vi "Drivetrain Loop.vi"() -> ()   [LabVIEW 2013]
uses:
  DT Mode.ctl
  Drivetrain Status.ctl
  Common Code/Change Detect Int.vi
  Robot Global Data.vi
  <vilib>/Rock Robotics/WPI/Solenoid/Deprecated/WPI_SolenoidSetBool.vi
  <vilib>/Rock Robotics/WPI/AnalogModule/WPI_AnalogModuleGetAverageVoltage.vi
  <vilib>/Utility/error.llb/Clear Errors.vi
panel:
  out "Mode":T1
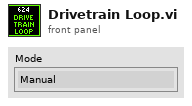
[diagram p1: front panel]
types:
  T1 = typedef "DT Mode.ctl" = enum16{"Manual", "Gyro Steer", "Distance Drive", "Fieldcentric", "Roll Maneuver", "Alt Roll Maneuver"}
  T2 = typedef "Drivetrain Status.ctl" = cluster{"Mode":T1, "X":dbl, "Y":dbl, "Steer":dbl, "Low Gear":bool, "Omni":bool}
  T3 = typedef "Drivetrain Control.ctl" = cluster{"axis 1 (x)":dbl, "axis 2 (y)":dbl, "Mode":T1, "heading target":dbl, "steer axis":dbl, "omni?":bool, "Low Gear?":bool, "distance target":cluster{"x":dbl, "y":dbl}, "PID Params":cluster{"X Dist":cluster{"PID gains":cluster{"proportional gain (Kc)":dbl, "integral time (Ti, min)":dbl, "derivative time (Td, min)":dbl}, "output range":cluster{"output high":dbl, "output low":dbl}}, "Y Dist":cluster{"PID gains":cluster{"proportional gain (Kc)":dbl, "integral time (Ti, min)":dbl, "derivative time (Td, min)":dbl}, "output range":cluster{"output high":dbl, "output low":dbl}}}, "Coast":bool}
  T4 = typedef "WPI_DriverStationRobotMode2.ctl" = enum16{"Autonomous Disabled", "Autonomous Enabled", "Teleop Disabled", "Teleop Enabled", "Timeout", "Finish", "Test Disabled", "Test Enabled"}
  T5 = typedef "Dashboard UDP Packet.ctl" = cluster{"Camera":T6, "Gyro":T7, "Encoder":T9, "Auto Shift":T10, "Auton":T11, "Drive/Ramp X":dbl, "Drive/Ramp Y":dbl, "Drive/Battery Cutoff":dbl, "Pressure/Compressor Min Voltage":dbl, "Pressure/Compressor Delay":dbl, "Controller/Strafe Correction":bool, "Shooter":T12, "Rollers":T13, "Abort":bool, "Finish":bool, "IR Halo Sustain Time":dbl, "Disable Compressor":bool, "Center Omni Drive Delay":i32, "Vision Mode":T14, "Radius Throttle":bool, "Fieldcentric":T15, "Roll":T16, "Stick Deadband":dbl}
  T6 = typedef "Camera Controls.ctl" = cluster{"Camera/View Angle X":dbl, "Camera/Goal Track Timeout":dbl, "Camera/View Angle Y":dbl, "Camera/Goal Exposure":dbl, "Camera/Vision Receive Timeout":dbl, "Camera/Offset 1":dbl, "Camera/Offset 2":dbl}
  T7 = typedef "Gyro Controls.ctl" = cluster{"Gyro/Angle Tolerance":dbl, "Gyro/Steer Closeness Threshold":dbl, "Steer PID":T8, "Steer Close PID":T8}
  T8 = typedef "PID Params.ctl" = cluster{"max":dbl, "min":dbl, "P":dbl, "I":dbl, "D":dbl}
  T9 = typedef "Encoder Controls.ctl" = cluster{"Encoders/Reset":bool, "Encoders/Omni Constant":dbl, "Encoders/Omni Tick Constant":dbl, "Encoders/Left Constant":dbl, "Encoders/Right Constant":dbl, "Encoders/Right Tick Constant":dbl}
  T10 = typedef "Auto Shift Controls.ctl" = cluster{"AutoShift/Upshift Throttle Accel":dbl, "AutoShift/Speed Threshold":dbl, "AutoShift/Upshift Throttle":dbl, "AutoShift/Upshift Accel":dbl, "AutoShift/Downshift Accel":dbl, "AutoShift/Downshift Throttle":dbl, "AutoShift/Delay":dbl, "AutoShift/Enabled":bool}
  T11 = typedef "Auton Controls.ctl" = cluster{"Auton/Left Shoot X-Coord":dbl, "Auton/Right Shoot X-Coord":dbl, "DistDrive/Distance Stop Threshold":dbl, "DistDrive/Max Stop Speed":dbl, "Auton/Back Piston Time":dbl, "Auton/Manual Hot":bool, "Auton/Manual Hot Right":bool, "Default X PID":T8, "Default Y PID":T8}
  T12 = typedef "Shooter Controls.ctl" = cluster{"Shooter/Reset Time":dbl, "Shooter/Release Delay":dbl, "Shooter/Pressure Steady Time":dbl, "Shooter/Misfire Delay":dbl, "Shooter/Ball Settle Time":dbl, "Shooter/Line IR Delay":dbl, "Pressure/Upper PSI Time":dbl, "Pressure/Lower PSI Time":dbl, "Shooter/Punch Delay":dbl, "Shooter/Target Pressure":dbl, "Pressure/Line B":dbl, "Pressure/Line M":dbl, "Pressure/Shooter M":dbl, "Pressure/Shooter B":dbl, "Halo Time":dbl, "Soft Release Delay":dbl, "Soft Unpin Delay":dbl, "Soft Shoot Delay":dbl}
  T13 = typedef "Roller Controls.ctl" = cluster{"Roller/Load IRs Verify Time":dbl, "Roller/Center IR Latch Time":dbl, "Roller/Speed Front":dbl, "Roller/Speed Back":dbl, "Roller/Entry Timeout":dbl, "Roller/To Center Timeout":dbl, "Roller/Sustain Time":dbl, "Roller/Verify Center Time":dbl}
  T14 = typedef "Vision Mode.ctl" = enum16{"Normal", "Extreme Left", "Extreme Right"}
  T15 = typedef "Fieldcentric Controls.ctl" = cluster{"Relative Angle":bool, "Point Robot":bool, "X/Y ratio low":dbl, "Steering Gain":dbl, "Force Omni Down":bool, "Enable":bool, "X/Y ratio high":dbl}
  T16 = typedef "Roll Maneuver.ctl" = cluster{"X 1":dbl, "Y 1":dbl, "Y 2":dbl, "X 2":dbl, "Y 3":dbl, "X 3":dbl, "Time 1":i32, "Time 2":i32, "Time 3":i32, "Angle Start":dbl, "Angle End":dbl, "Angle Linearity":dbl}
  T17 = cluster{"X Dist":cluster{"PID gains":cluster{"proportional gain (Kc)":dbl, "integral time (Ti, min)":dbl, "derivative time (Td, min)":dbl}, "output range":cluster{"output high":dbl, "output low":dbl}}, "Y Dist":cluster{"PID gains":cluster{"proportional gain (Kc)":dbl, "integral time (Ti, min)":dbl, "derivative time (Td, min)":dbl}, "output range":cluster{"output high":dbl, "output low":dbl}}}
  T18 = typedef "WPI_SolenoidDevRef.ctl" = cluster{"DevStatus":errorcluster, "Solenoid Module":T19, "Forward Solenoid Channel":T20, "Reverse Solenoid Channel":T20}
  T19 = typedef "FPGA_TypedefSolenoidModule.ctl" = enum16{"Solenoid Module 1", "Solenoid Module 2"}
  T20 = typedef "WPI_SolenoidChannel.ctl" = enum8{"Solenoid 1", "Solenoid 2", "Solenoid 3", "Solenoid 4", "Solenoid 5", "Solenoid 6", "Solenoid 7", "Solenoid 8", "Invalid"}
  T21 = typedef "WPI_MotorControlDeviceRef.ctl" = cluster{"DeviceStatus":errorcluster, "Type":enum16{"PWM", "CAN"}, "PWM":cluster{"Digital Module":T22, "PWM Channel":T23, "DeadBand":T24}, "CAN":cluster{"Device Number":u8, "Control Mode":T25, "Semaphore":T26, "Max Vout":dbl}, "Invert":bool, "TransformRef":T27, "InvTransformRef":T27}
  T22 = typedef "FPGA_TypedefDigitalModule.ctl" = enum16{"Digital Module 1", "Digital Module 2"}
  T23 = typedef "FPGA_DIOPWMChannel.ctl" = enum8{"PWM 1", "PWM 2", "PWM 3", "PWM 4", "PWM 5", "PWM 6", "PWM 7", "PWM 8", "PWM 9", "PWM 10", "Invalid"}
  T24 = typedef "WPI_PWMDeadband.ctl" = cluster{"Name":string, "maxPositivePwm":i32, "minPositivePwm":i32, "centerPwm":i32, "maxNegativePwm":i32, "minNegativePwm":i32, "angularRange":u16}
  T25 = typedef "WPI_CANJaguar_ControlMode.ctl" = enum8{"Percent VBus", "Current", "Speed", "Position", "Voltage"}
  T26 = typedef "Semaphore RefNum" = refnum<k1>
  T27 = typedef "WPI_PWMTransform_ConPane.ctl" = refnum<vi>
  T28 = typedef "Arcade Drive Ref.ctl" = cluster{"L1":T21, "L2":T21, "R1":T21, "R2":T21, "Motor Count":enum16{"2 Motor", "4 Motor"}, "L Reversed?":bool, "R Reversed?":bool}
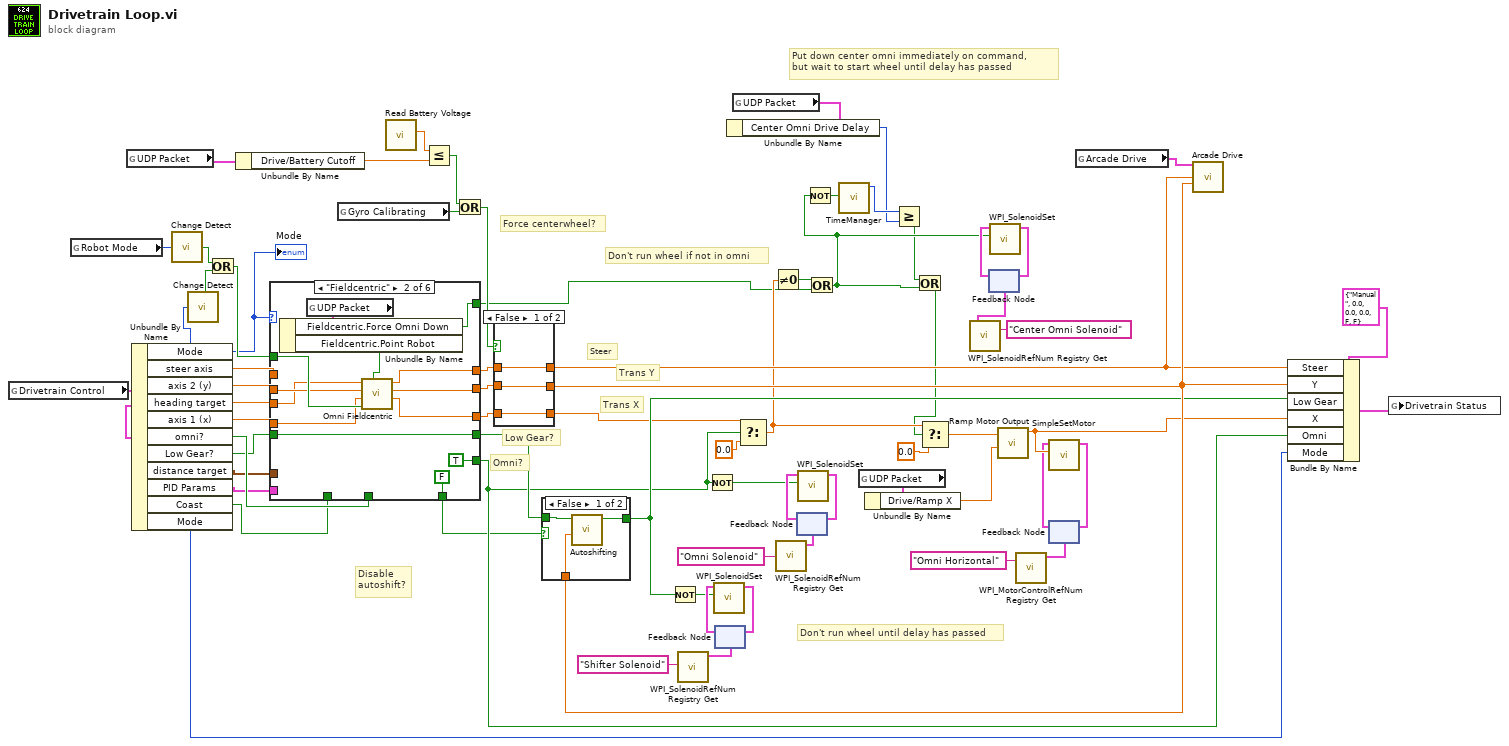
[diagram p0: block diagram]
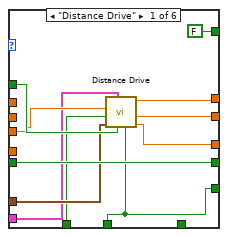
[diagram p3: hidden frame]
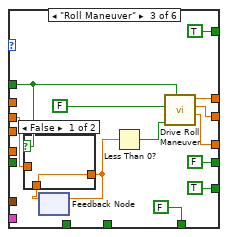
[diagram p4: hidden frame]
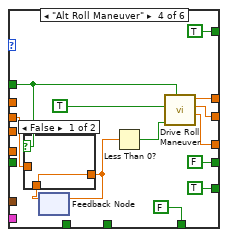
[diagram p6: hidden frame]
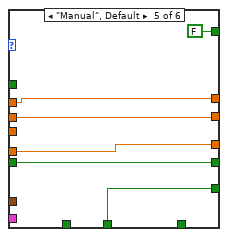
[diagram p8: hidden frame]
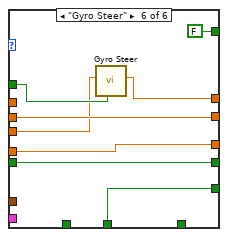
[diagram p9: hidden frame]
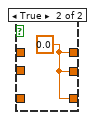
[diagram p10: hidden frame]
diagram:
  # "Disable \nautoshift?"
  # "Force centerwheel?"
  # "Don't run wheel until delay has passed"
  # "Don't run wheel if not in omni"
  # "Put down center omni immediately on command,\nbut wait to start wheel until delay has passed"
  # "Low Gear?"
  # "Omni?"
  # "Trans X"
  # "Steer"
  # "Trans Y"
  n1 = global read "Robot Global Data.vi" "Drivetrain Control"() -> (w51:T3)
  n2 = global read "Robot Global Data.vi" "Robot Mode"() -> (w67:T4)
  n3 = global read "Robot Global Data.vi" "UDP Packet"() -> (w45:T5)
  n4 = Unbundle By Name(w51) -> ("Mode"=w60:T1, "steer axis"=w59:dbl, "axis 2 (y)"=w58:dbl, "heading target"=w57:dbl, "axis 1 (x)"=w56:dbl, "omni?"=w55:bool, "Low Gear?"=w54:bool, "distance target"=w53:cluster{"x":dbl, "y":dbl}, "PID Params"=w52:T17, "Coast"=w46:bool, "Mode"=w1:T1)
  "Mode" <- w60
  n5 = call-poly "Change Detect.vi"("In"=w67) -> ("Changed?"=w68:bool)
  n6 = call-poly "Change Detect.vi"("In"=w60) -> ("Changed?"=w69:bool)
  n7 = Or(x=w68, y=w69) -> (x .or. y?=w63:bool)
  n8 = Unbundle By Name(w45) -> ("Drive/Battery Cutoff"=w44:dbl)
  n9 = case shown="\"Fieldcentric\"" w60 {
    tunnel: w59 -> [_ _ _ _ w129 _]
    tunnel: [w76 w87 w106 w121 w129 w133] -> w66
    tunnel: w58 -> [_ w91 w97 w112 w128 w137]
    tunnel: [w77 w88 w105 w120 w128 w137] -> w65
    tunnel: w63 -> [w75 w93 w98 w113 _ w132]
    tunnel: w57 -> [w74 w90 _ _ _ w131]
    tunnel: [w78 w89 w104 w119 w127 w136] -> w64
    tunnel: w56 -> [_ w92 _ _ w127 w136]
    tunnel: w55 -> [w79 _ _ _ w125 w134]
    tunnel: w54 -> [w80 w81 _ _ w126 w135]
    tunnel: w52 -> [w72 _ _ _ _ _]
    tunnel: w53 -> [w73 _ _ _ _ _]
    tunnel: [w80 w81 FALSE ("Low Gear?") FALSE ("Low Gear?") w126 w135] -> w62
    tunnel: [w79 TRUE ("omni?") TRUE ("omni?") TRUE ("omni?") w125 w134] -> w20
    tunnel: w46 -> [w71 _ _ _ _ _]
    tunnel: [FALSE w84 TRUE ("Force Omni Down") TRUE ("Force Omni Down") FALSE FALSE] -> w6
    tunnel: [_ FALSE ("Force Omni Down") FALSE ("Force Omni Down") FALSE ("Force Omni Down") _ _] -> w2
    frame "Distance Drive" {
      n10 = call "Distance Drive.vi"("omni?"=w79, "reinit?"=w75, "PID Params"=w72, "distance target"=w73, "coast?"=w71, "Heading"=w74) -> ("X"=w78:dbl, "Y"=w77:dbl, "X steer"=w76:dbl)  [unwired: 3 in]
    }
    frame "Fieldcentric" {
      n11 = global read "Robot Global Data.vi" "UDP Packet"() -> (w85:T5)
      n12 = Unbundle By Name(w85) -> ("Fieldcentric.Force Omni Down"=w84:bool, "Fieldcentric.Point Robot"=w83:bool)
      n13 = call "Omni Fieldcentric.vi"("Point Robot"=w83, "reinit?"=w93, "axis 1 (x)"=w92, "axis 2 (y)"=w91, "Steer Target Angle"=w90) -> ("Translation X"=w89:dbl, "Translation Y"=w88:dbl, "Rotation"=w87:dbl)  [unwired: 4 in]
    }
    frame "Roll Maneuver" {
      n14 = feedback #1() -> (w96:dbl)  [unwired: 1 in]
      n15 = case shown="False" w98 {
        tunnel: w97 -> [_ w108]
        tunnel: [w107 w108] -> w95
        tunnel: w96 -> [w107 _]
        frame False {
        }
        frame True {
        }
      }
      n16 = feedback-in #1(w95) -> ()
      n17 = Less Than 0?(x=w95) -> (x < 0?=w94:bool)
      n18 = call "Drive Roll Maneuver.vi"("Reset?"=w98, "Backwards?"=w94, "Alt Side"=FALSE) -> ("X"=w104:dbl, "Y"=w105:dbl, "Steer"=w106:dbl)  [unwired: 6 in]
    }
    frame "Alt Roll Maneuver" {
      n19 = feedback #2() -> (w111:dbl)  [unwired: 1 in]
      n20 = case shown="False" w113 {
        tunnel: w112 -> [_ w123]
        tunnel: [w122 w123] -> w110
        tunnel: w111 -> [w122 _]
        frame False {
        }
        frame True {
        }
      }
      n21 = feedback-in #2(w110) -> ()
      n22 = Less Than 0?(x=w110) -> (x < 0?=w109:bool)
      n23 = call "Drive Roll Maneuver.vi"("Reset?"=w113, "Backwards?"=w109, "Alt Side"=TRUE) -> ("X"=w119:dbl, "Y"=w120:dbl, "Steer"=w121:dbl)  [unwired: 6 in]
    }
    frame "Manual", Default {
    }
    frame "Gyro Steer" {
      n24 = call "Gyro Steer.vi"("reinitialize? (F)"=w132, "Target Angle"=w131) -> ("Steering Out"=w133:dbl)  [unwired: 8 in, 1 out]
    }
  }
  n25 = global read "Robot Global Data.vi" "Gyro Calibrating"() -> (w50:bool)
  n26 = call "Read Battery Voltage.vi"() -> ("Voltage"=w48:dbl)  [unwired: 11 in]
  n27 = Less Or Equal?(x=w48, y=w44) -> (x <= y?=w47:bool)
  n28 = Or(x=w47, y=w50) -> (x .or. y?=w49:bool)
  n29 = case shown="False" w49 {
    tunnel: w66 -> [w140 _]
    tunnel: [w140 w141] -> w41
    tunnel: w65 -> [w139 _]
    tunnel: [w139 w141] -> w43
    tunnel: w64 -> [w138 _]
    tunnel: [w138 w141] -> w15
    frame False {
    }
    frame True {
      w141 = 0.0 ("Rotation")
    }
  }
  n30 = case shown="False" w2 {
    tunnel: w62 -> [w144 w145]
    tunnel: w43 -> [w143 _]
    tunnel: [w142 w145] -> w23
    frame False {
      n31 = call "Autoshifting.vi"("Throttle"=w143, "Manual Low Gear"=w144) -> ("Low Gear"=w142:bool)  [unwired: 9 in]
    }
    frame True {
    }
  }
  n32 = Not(x=w23) -> (.not. x?=w28:bool)
  n33 = call <vilib>:"WPI_SolenoidRefNum Registry Get.vi"("refnum name"="Shifter Solenoid") -> ("SolenoidDevRef"=w32:T18)  [unwired: 9 in, 1 out]
  n34 = Not(x=w20) -> (.not. x?=w29:bool)
  n35 = feedback #3(w32) -> (w30:T18)
  n36 = call-poly <vilib>:"WPI_SolenoidSet.vi"("Value"=w28, "SolenoidDevRef"=w30) -> ("SolenoidDevRef"=w33:T18)  [unwired: 8 in, 1 out]
  n37 = feedback-in #3(w33) -> ()
  n38 = global read "Robot Global Data.vi" "UDP Packet"() -> (w12:T5)
  n39 = Unbundle By Name(w12) -> ("Center Omni Drive Delay"=w11:i32)
  n40 = Select(t=w15, s=w20, f=0.0) -> (s? t:f=w8:dbl)
  n41 = Not Equal To 0?(x=w8) -> (x != 0?=w7:bool)
  n42 = call <vilib>:"WPI_SolenoidRefNum Registry Get.vi"("refnum name"="Omni Solenoid") -> ("SolenoidDevRef"=w37:T18)  [unwired: 9 in, 1 out]
  n43 = feedback #4(w37) -> (w36:T18)
  n44 = call-poly <vilib>:"WPI_SolenoidSet.vi"("Value"=w29, "SolenoidDevRef"=w36) -> ("SolenoidDevRef"=w35:T18)  [unwired: 8 in, 1 out]
  n45 = feedback-in #4(w35) -> ()
  n46 = Or(x=w7, y=w6) -> (x .or. y?=w5:bool)
  n47 = Not(x=w5) -> (.not. x?=w14:bool)
  n48 = call "TimeManager.vi"("Reset?"=w14) -> ("Time Since Reset"=w13:u32)  [unwired: 9 in, 1 out]
  n49 = global read "Robot Global Data.vi" "UDP Packet"() -> (w25:T5)
  n50 = Unbundle By Name(w25) -> ("Drive/Ramp X"=w24:dbl)
  n51 = Greater Or Equal?(x=w13, y=w11) -> (x >= y?=w4:bool)
  n52 = Or(x=w4, y=w5) -> (x .or. y?=w3:bool)
  n53 = Select(t=w8, s=w3, f=0.0) -> (s? t:f=w9:dbl)
  n54 = call <vilib>:"WPI_SolenoidRefNum Registry Get.vi"("refnum name"="Center Omni Solenoid") -> ("SolenoidDevRef"=w18:T18)  [unwired: 9 in, 1 out]
  n55 = feedback #5(w18) -> (w17:T18)
  n56 = call-poly <vilib>:"WPI_SolenoidSet.vi"("Value"=w5, "SolenoidDevRef"=w17) -> ("SolenoidDevRef"=w16:T18)  [unwired: 8 in, 1 out]
  n57 = feedback-in #5(w16) -> ()
  n58 = call "Ramp Motor Output.vi"("Ramp Time"=w24, "Input"=w9) -> ("Output"=w42:dbl)  [unwired: 9 in]
  n59 = call <vilib>:"WPI_MotorControlRefNum Registry Get.vi"("refnum name"="Omni Horizontal") -> ("MotorControlDevRef"=w40:T21)  [unwired: 9 in, 1 out]
  n60 = feedback #6(w40) -> (w26:T21)
  n61 = call "SimpleSetMotor.vi"("Output"=w42, "MotorControlDevRef"=w26) -> ("MotorControlDevRef"=w27:T21)  [unwired: 8 in, 1 out]
  n62 = feedback-in #6(w27) -> ()
  n63 = global read "Robot Global Data.vi" "Arcade Drive"() -> (w61:T28)
  n64 = call "Arcade Drive.vi"("Ref In"=w61, "X"=w41, "Y"=w43) -> ()  [unwired: 13 in]
  n65 = Bundle By Name(cluster=T2 {"Mode"=enum."Manual", "X"=0.0, "Y"=0.0, "Steer"=0.0, "Low Gear"=FALSE, "Omni"=FALSE} ("Drivetrain Status"), "Steer"=w41, "Y"=w43, "Low Gear"=w23, "X"=w42, "Omni"=w20, "Mode"=w1) -> (w21:T2)
  n66 = global write "Robot Global Data.vi" "Drivetrain Status"(w21) -> ()
